vi "Generate Error.vi"(7 "Is Warning? (False)":bool, 8 "Error In":errorcluster, 9 "Arguments":string[](array[string]), 10 "Error Type":T5, 11 "LINX Device Config":T1) -> (0 "Error Out":errorcluster, 3 "Dup LINX Device Config":T1)   [LabVIEW 2014, in "LMH-LINX.lvlib"]
doc: "Generate a LINX error based on the Error Type input."
uses:
  <vilib>/MakerHub/LINX/LMH-LINX.lvlib
  <vilib>/MakerHub/LINX/Private/Type Defs/Error Type.ctl
  <vilib>/MakerHub/LINX/Private/Device/Type Defs/LINX Device Config.ctl
  <vilib>/MakerHub/LINX/Private/Type Defs/Interface.ctl
  <vilib>/MakerHub/LINX/Private/Device/Type Defs/TCP Config.ctl
  <vilib>/MakerHub/LINX/Private/Device/Type Defs/Channels.ctl
  <vilib>/MakerHub/LINX/Private/Device/Device.lvlib
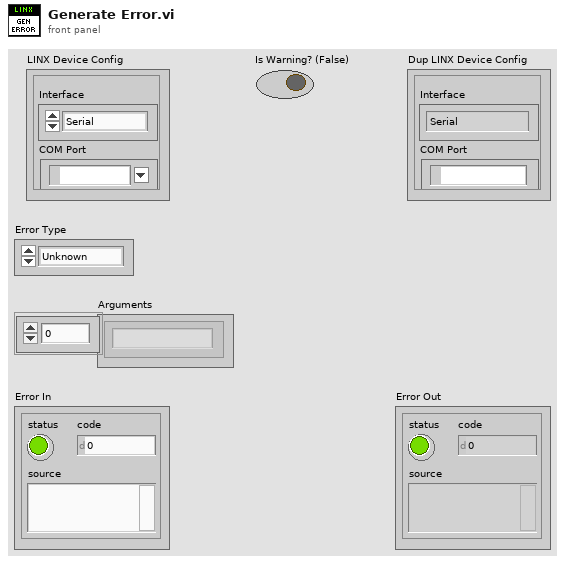
[diagram p1: front panel]
types:
  T1 = typedef "LMH-LINX.lvlib/Device.lvlib/LINX Device Config.ctl" = cluster{"Interface":T2, "COM Port":refnum<visa-resource-name>, "TCP Configuration":T3, "Device Family":u8, "Device ID":u8, "Device Name":string, "TCP Ref":refnum<k5>, "Channels":T4}
  T2 = typedef "LMH-LINX.lvlib/Interface.ctl" = enum16{"Serial", "TCP"}
  T3 = typedef "LMH-LINX.lvlib/Device.lvlib/TCP Config.ctl" = cluster{"IP Address":string, "Port":u16}
  T4 = typedef "LMH-LINX.lvlib/Channels.ctl" = cluster{"DI":u8[], "DO":u8[], "AI":u8[], "AO":u8[], "PWM":u8[], "QE":u8[], "UART":u8[], "I2C 2":u8[], "SPI":u8[], "CAN":u8[], "Servo":u8[], "AI Ref (V)":dbl, "AO Ref (V)":dbl, "AO Resolution (Bits)":u8}
  T5 = typedef "LMH-LINX.lvlib/Error Type.ctl" = enum16{"Unknown", "Timeout", "Corrupt Return Packet", "Unable To Connect", "Command Not Supported", "Channel DNE", "Invalid COM Config", "Firmware Version Mismatch", "myRIO Support", "CMD Specific Error", "Local IO Not Supported"}
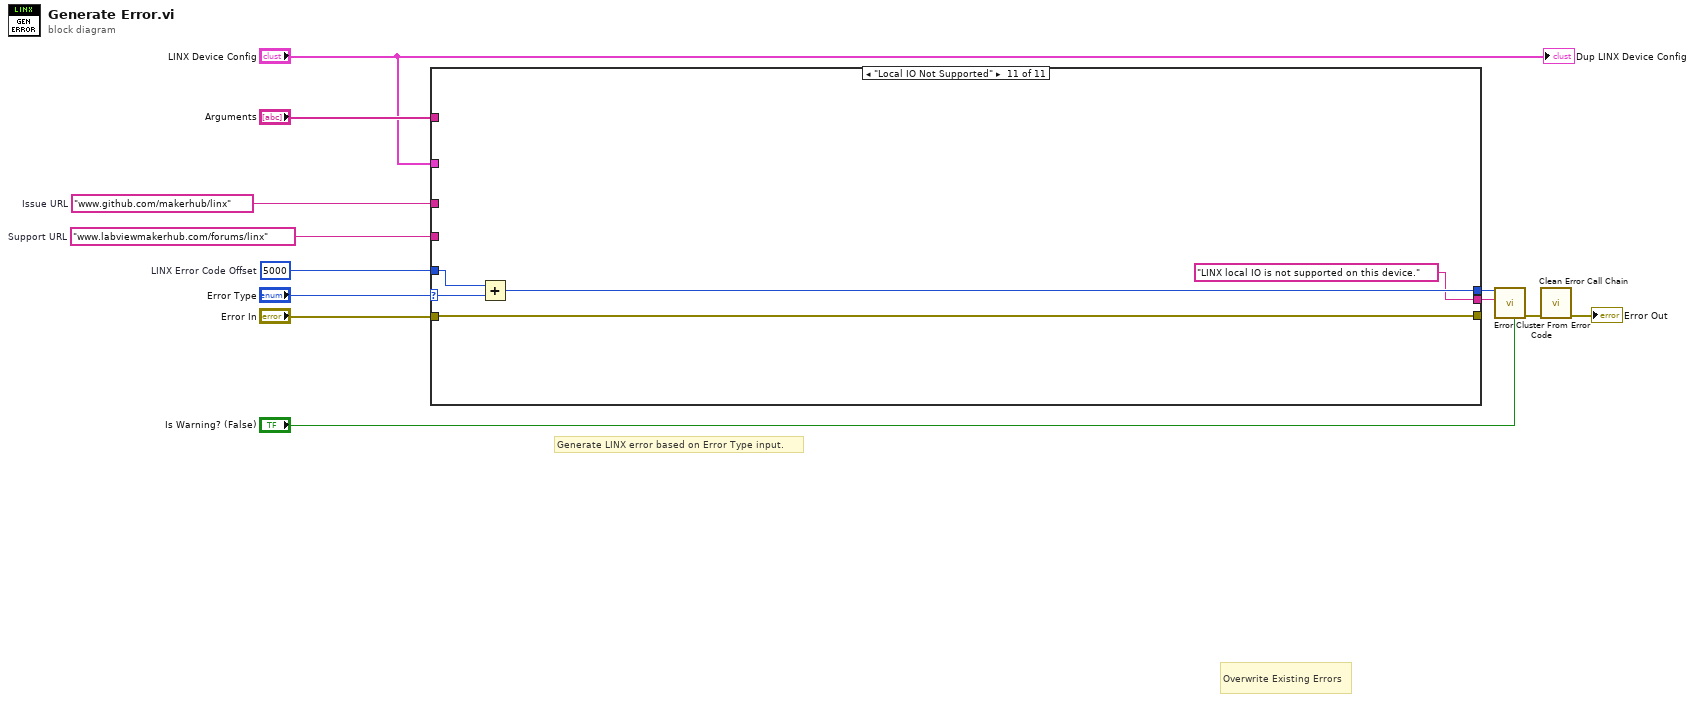
[diagram p0: block diagram]
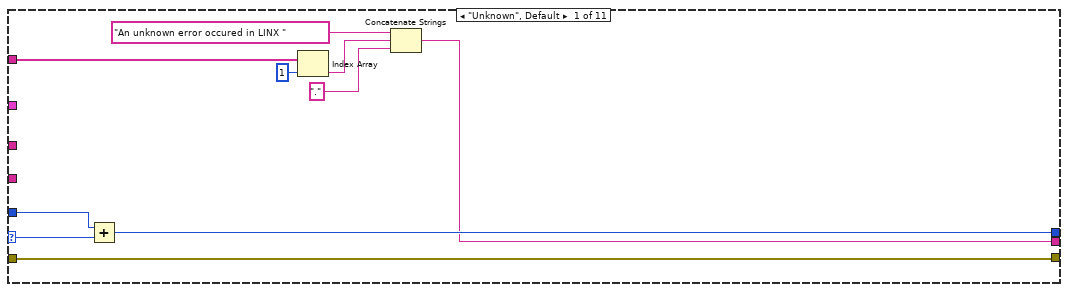
[diagram p2: hidden frame]
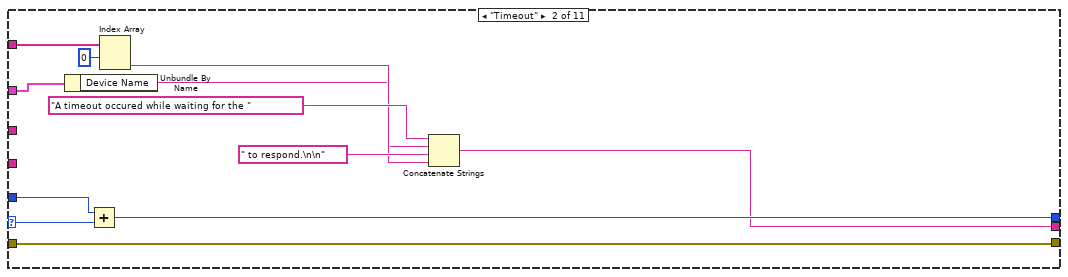
[diagram p3: hidden frame]
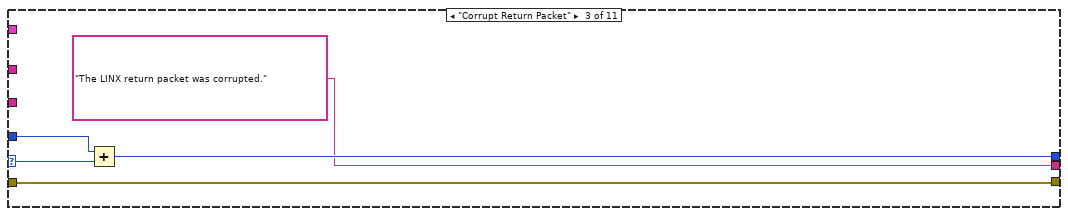
[diagram p4: hidden frame]
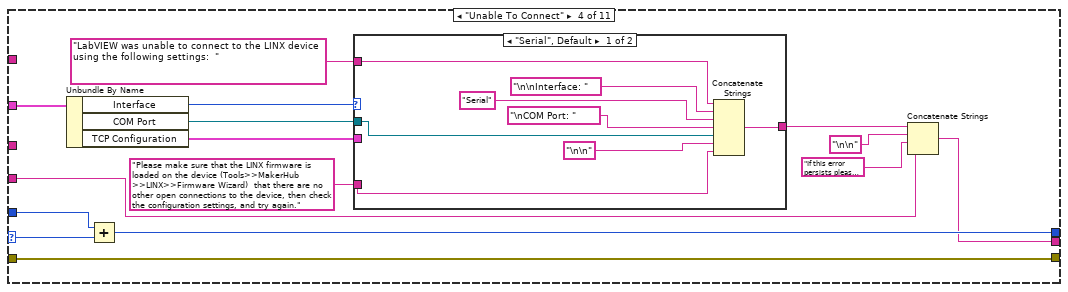
[diagram p5: hidden frame]
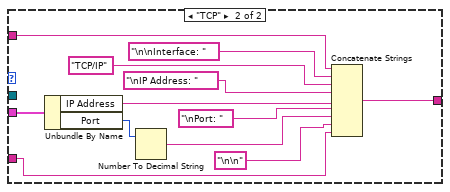
[diagram p6: hidden frame]
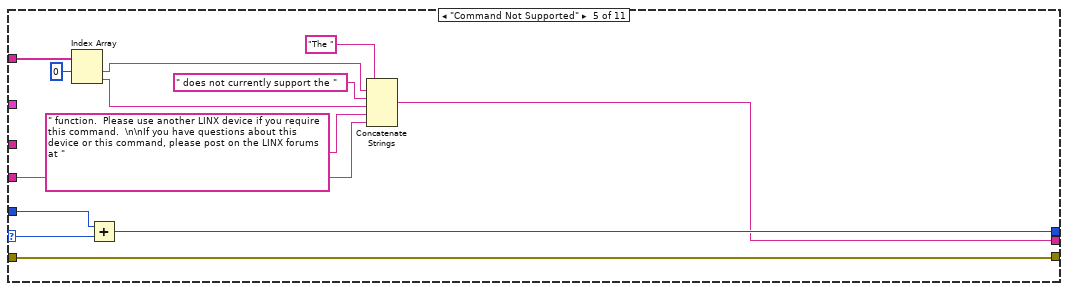
[diagram p7: hidden frame]
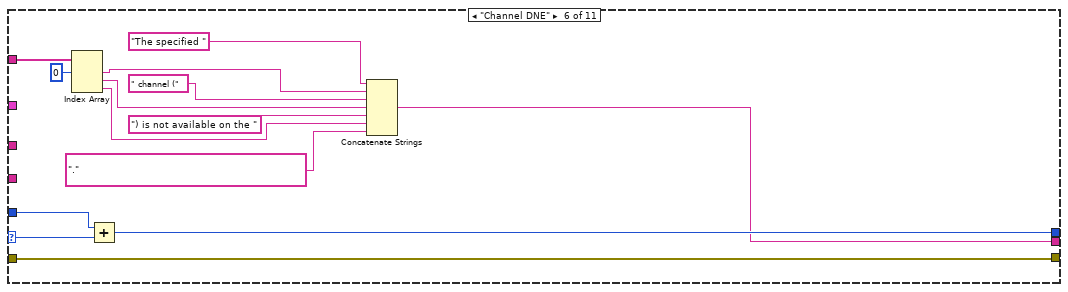
[diagram p8: hidden frame]
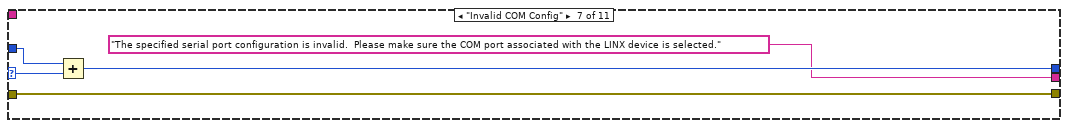
[diagram p9: hidden frame]
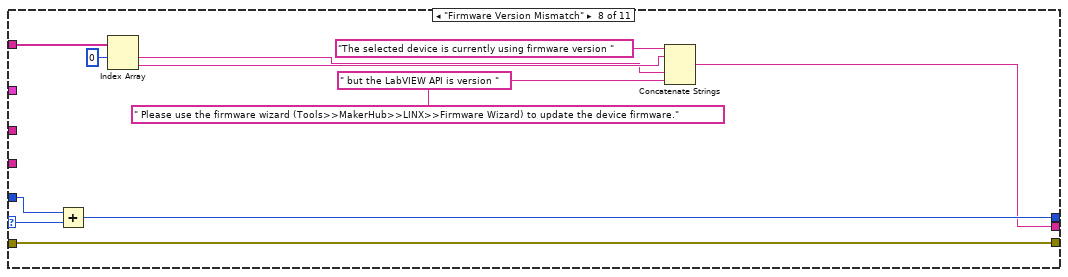
[diagram p10: hidden frame]
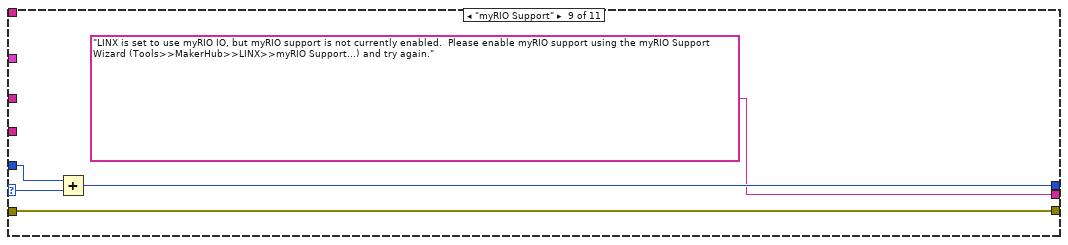
[diagram p11: hidden frame]
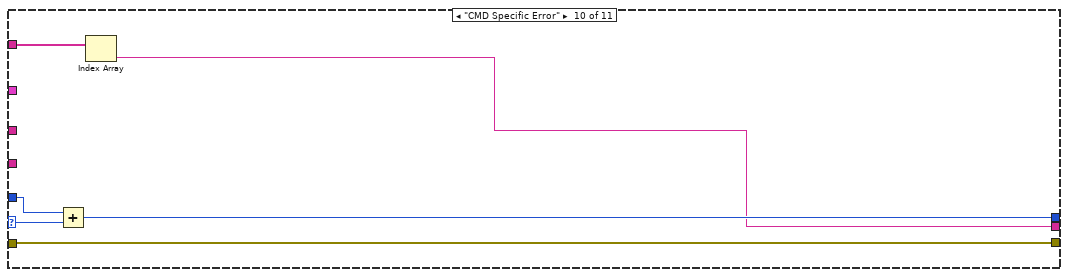
[diagram p12: hidden frame]
diagram:
  w3 = "www.labviewmakerhub.com/forums/linx"  # Support URL
  w6 = "www.github.com/makerhub/linx"  # Issue URL
  w11 = 5000  # LINX Error Code Offset
  # "Overwrite Existing Errors"
  # "Generate LINX error based on Error Type input."
  n1 = case shown="\"Local IO Not Supported\"" "Error Type" {
    selector: "Error Type" -> [w21 w33 w38 w53 w86 w100 w105 w117 w122 w128 w133]
    tunnel: "Error In" -> [w20 w31 w35 w52 w85 w99 w102 w115 w120 w126 w131]
    tunnel: [w20 w31 w35 w52 w85 w99 w102 w115 w120 w126 w131] -> _
    tunnel: w11 -> [w22 w34 w39 w54 w87 w101 w106 w118 w123 w129 w134]
    tunnel: [w14 w29 "The LINX return packet was corrupted." ("error message (\"\")") w41 w81 w97 "The specified serial port configuration is invalid.  Please make sure the COM port associated with the LINX device is selected." w107 "LINX is set to use myRIO IO, but myRIO support is not currently enabled.  Please enable myRIO support using the myRIO Support Wizard (Tools>>MakerHub>>LINX>>myRIO Support...) and try again." ("Issue URL") w124 "LINX local IO is not supported on this device." ("Arguments")] -> w9
    tunnel: [w19 w32 w37 w51 w84 w98 w104 w116 w121 w127 w132] -> w8
    tunnel: w6 -> [_ _ _ _ _ _ _ _ _ _ _]
    tunnel: "Arguments" -> [w17 w28 _ _ w79 w96 _ w114 _ w125 _]
    tunnel: "LINX Device Config" -> [_ w24 _ w50 _ _ _ _ _ _ _]
    tunnel: w3 -> [_ _ _ w40 w76 _ _ _ _ _ _]
    frame "Unknown", Default {
      n2 = Add(x=w22, y=w21) -> (x+y=w19:i32)
      n3 = Index Array(array=w17, index=1) -> (element=w16:string)
      n4 = Concatenate Strings("An unknown error occured in LINX " ("error message (\"\")"), w16, "." ("string")) -> (w14:string)
    }
    frame "Timeout" {
      n5 = Unbundle By Name(w24) -> ("Device Name"=w23:string)
      n6 = Add(x=w34, y=w33) -> (x+y=w32:i32)
      n7 = Index Array(array=w28, index #1=0 ("index")) -> (element #2=w25:string)  [unwired: 1 in, 1 out]
      n8 = Concatenate Strings("A timeout occured while waiting for the " ("error message (\"\")"), w23, " to respond.\n\n" ("string"), w25) -> (w29:string)
    }
    frame "Corrupt Return Packet" {
      n9 = Add(x=w39, y=w38) -> (x+y=w37:i32)
    }
    frame "Unable To Connect" {
      n10 = Unbundle By Name(w50) -> ("Interface"=w49:T2, "COM Port"=w45:refnum<visa-resource-name>, "TCP Configuration"=w48:T3)
      n11 = Add(x=w54, y=w53) -> (x+y=w51:i32)
      n12 = case shown="\"Serial\", Default" w49 {
        tunnel: w48 -> [_ w74]
        tunnel: "LabVIEW was unable to connect to the LINX device using the following settings:  " ("error message (\"\")") -> [w59 w70]
        tunnel: "Please make sure that the LINX firmware is loaded on the device (Tools>>MakerHub >>LINX>>Firmware Wizard)  that there are no other open connections to the device, then check the configuration settings, and try again." -> [w55 w64]
        tunnel: [w57 w63] -> w44
        tunnel: w45 -> [w58 _]
        frame "Serial", Default {
          n13 = Concatenate Strings(w59, "\n\nInterface: " ("string"), "Serial" ("string"), "\nCOM Port: " ("string"), w58, "\n\n" ("string"), w55) -> (w57:string)
        }
        frame "TCP" {
          n14 = Unbundle By Name(w74) -> ("IP Address"=w68:string, "Port"=w73:u16)
          n15 = Number To Decimal String(number=w73) -> (decimal integer string=w66:string)  [unwired: 1 in]
          n16 = Concatenate Strings(w70, "\n\nInterface: " ("string"), "TCP/IP" ("string"), "\nIP Address: " ("string"), w68, "\nPort: " ("string"), w66, "\n\n" ("string"), w64) -> (w63:string)
        }
      }
      n17 = Concatenate Strings(w44, "\n\n" ("string"), "If this error persists please search, then post on the LINX forums at " ("error message (\"\")"), w40) -> (w41:string)
    }
    frame "Command Not Supported" {
      n18 = Index Array(array=w79, index #1=0 ("index")) -> (element #1=w75:string, element #2=w77:string)  [unwired: 1 in]
      n19 = Add(x=w87, y=w86) -> (x+y=w84:i32)
      n20 = Concatenate Strings("The " ("string"), w75, " does not currently support the " ("string"), w77, " function.  Please use another LINX device if you require this command.  \n\nIf you have questions about this device or this command, please post on the LINX forums at " ("string"), w76) -> (w81:string)
    }
    frame "Channel DNE" {
      n21 = Index Array(array=w96, index #1=0 ("index")) -> (element #1=w94:string, element #2=w93:string, element #3=w89:string)  [unwired: 2 in]
      n22 = Add(x=w101, y=w100) -> (x+y=w98:i32)
      n23 = Concatenate Strings("The specified ", w94, " channel (" ("string"), w93, ") is not available on the " ("string"), w89, "." ("string")) -> (w97:string)
    }
    frame "Invalid COM Config" {
      n24 = Add(x=w106, y=w105) -> (x+y=w104:i32)
    }
    frame "Firmware Version Mismatch" {
      n25 = Add(x=w118, y=w117) -> (x+y=w116:i32)
      n26 = Index Array(array=w114, index #1=0 ("index")) -> (element #1=w109:string, element #2=w111:string)  [unwired: 1 in]
      n27 = Concatenate Strings("The selected device is currently using firmware version " ("Issue URL"), w111, " but the LabVIEW API is version " ("Issue URL"), w109, " Please use the firmware wizard (Tools>>MakerHub>>LINX>>Firmware Wizard) to update the device firmware." ("Issue URL")) -> (w107:string)
    }
    frame "myRIO Support" {
      n28 = Add(x=w123, y=w122) -> (x+y=w121:i32)
    }
    frame "CMD Specific Error" {
      n29 = Add(x=w129, y=w128) -> (x+y=w127:i32)
      n30 = Index Array(array=w125) -> (element=w124:string)  [unwired: 1 in]
    }
    frame "Local IO Not Supported" {
      n31 = Add(x=w134, y=w133) -> (x+y=w132:i32)
    }
  }
  n32 = call <vilib>:"Error Cluster From Error Code.vi"("is warning? (False)"="Is Warning? (False)", "error message (\"\")"=w9, "error code (0)"=w8) -> ("error out"=w2:errorcluster)  [unwired: 6 in]
  n33 = call <vilib>:"Clean Error Call Chain.vi"("Error In"=w2) -> ("Error Out"=→"Error Out":errorcluster)  [unwired: 10 in]
  "Dup LINX Device Config" <- "LINX Device Config"
